vi "Format Http Request.vi"(0 "WS URI":string="ws://hostname.domain:80/resource/name", 2 "header string in":string, 3 "WebSocket Key":string="dKP/0gJzWzXMAh6SYdQ/sA==", 5 "error in":errorcluster, 9 "Relative URI Request (F)":bool) -> (16 "Http Request":string, 19 "error out":errorcluster)   [LabVIEW 2021, in "LV WebSockets.lvlib"]
uses:
  LV WebSockets.lvlib
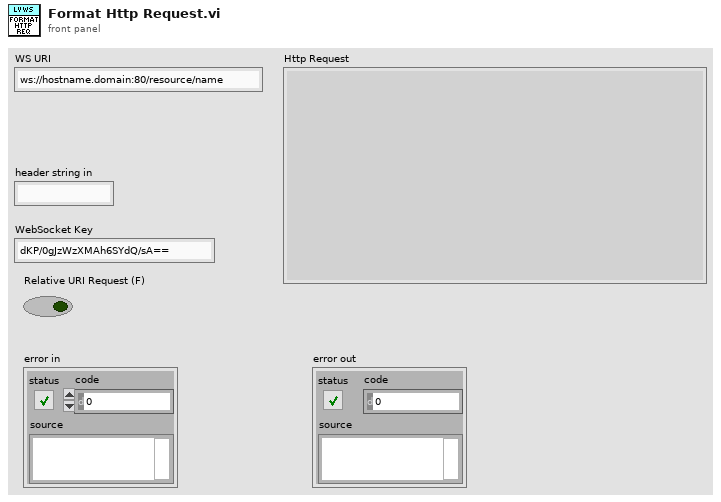
[diagram p1: front panel]
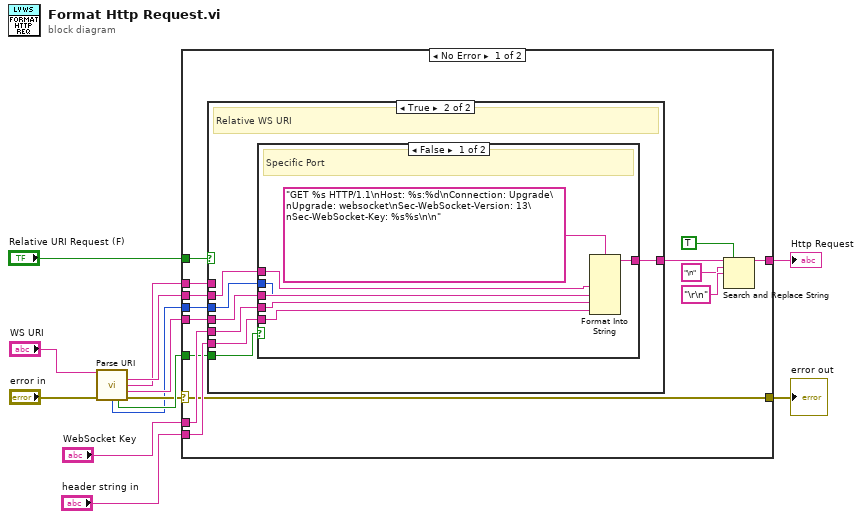
[diagram p0: block diagram]
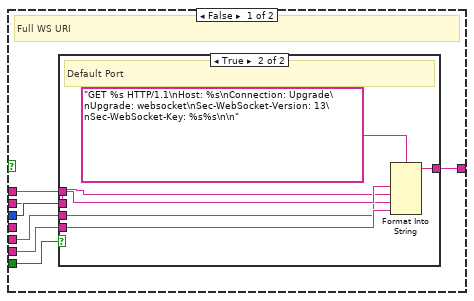
[diagram p2: hidden frame]
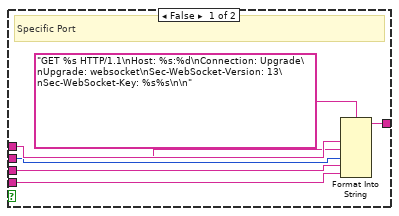
[diagram p3: hidden frame]
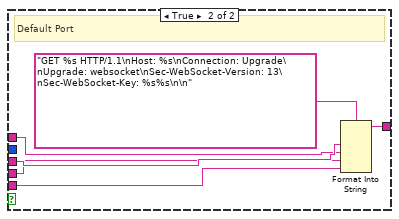
[diagram p4: hidden frame]
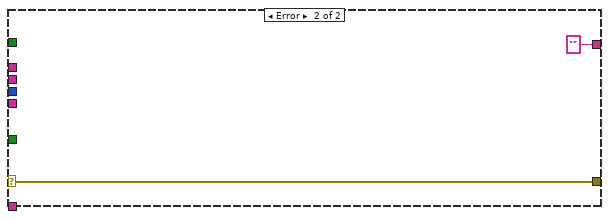
[diagram p5: hidden frame]
diagram:
  n1 = call "Parse URI.vi"("URI"="WS URI", "error in"="error in") -> ("Hostname"=w8:string, "HTTP URI"=w1:string, "Resource Name"=w3:string, "Port"=w2:u16, "Default Port"=w6:bool, "error out"=w5:errorcluster)  [unwired: 7 in, 1 out]
  n2 = case shown="No Error" w5 {
    selector: w5 -> [w15 w69]
    tunnel: "header string in" -> [w27 _]
    tunnel: "WebSocket Key" -> [w24 _]
    tunnel: [w22 "" ("result string")] -> w11
    tunnel: "Relative URI Request (F)" -> [w20 _]
    tunnel: w2 -> [w19 _]
    tunnel: w1 -> [w18 _]
    tunnel: w8 -> [w17 _]
    tunnel: w6 -> [w16 _]
    tunnel: [w15 w69] -> w4
    tunnel: w3 -> [w14 _]
    frame No Error {
      n3 = case shown="True" w20 {
        tunnel: w19 -> [w34 w50]
        tunnel: w18 -> [w33 _]
        tunnel: w27 -> [w32 w54]
        tunnel: w24 -> [w31 w53]
        tunnel: [w30 w52] -> w23
        tunnel: w17 -> [w28 w51]
        tunnel: w16 -> [w29 w49]
        tunnel: w14 -> [_ w48]
        frame False {
          # "Full WS URI"
          n4 = case shown="True" w29 {
            tunnel: w34 -> [w36 _]
            tunnel: w33 -> [w41 w47]
            tunnel: w32 -> [w40 w46]
            tunnel: w31 -> [w39 w45]
            tunnel: [w37 w43] -> w30
            tunnel: w28 -> [w35 w42]
            frame False {
              # "Specific Port"
              n5 = Format Into String(format string="GET %s HTTP/1.1\nHost: %s:%d\nConnection: Upgrade\nUpgrade: websocket\nSec-WebSocket-Version: 13\nSec-WebSocket-Key: %s%s\n\n", w41, w35, w36, w39, w40) -> (resulting string=w37:string)  [unwired: 2 in, 1 out]
            }
            frame True {
              # "Default Port"
              n6 = Format Into String(format string="GET %s HTTP/1.1\nHost: %s\nConnection: Upgrade\nUpgrade: websocket\nSec-WebSocket-Version: 13\nSec-WebSocket-Key: %s%s\n\n", w47, w42, w45, w46) -> (resulting string=w43:string)  [unwired: 2 in, 1 out]
            }
          }
        }
        frame True {
          # "Relative WS URI"
          n7 = case shown="False" w49 {
            tunnel: w48 -> [w61 w67]
            tunnel: w54 -> [w60 w66]
            tunnel: w53 -> [w59 w65]
            tunnel: [w57 w63] -> w52
            tunnel: w51 -> [w56 w62]
            tunnel: w50 -> [w55 _]
            frame False {
              # "Specific Port"
              n8 = Format Into String(format string="GET %s HTTP/1.1\nHost: %s:%d\nConnection: Upgrade\nUpgrade: websocket\nSec-WebSocket-Version: 13\nSec-WebSocket-Key: %s%s\n\n", w61, w56, w55, w59, w60) -> (resulting string=w57:string)  [unwired: 2 in, 1 out]
            }
            frame True {
              # "Default Port"
              n9 = Format Into String(format string="GET %s HTTP/1.1\nHost: %s\nConnection: Upgrade\nUpgrade: websocket\nSec-WebSocket-Version: 13\nSec-WebSocket-Key: %s%s\n\n", w67, w62, w65, w66) -> (resulting string=w63:string)  [unwired: 2 in, 1 out]
            }
          }
        }
      }
      n10 = Search and Replace String(replace all?=TRUE ("replace all? (F)"), input string=w23, search string="\n", replace string="\r\n" ("replace string (\"\")")) -> (result string=w22:string)  [unwired: 4 in, 3 out]
    }
    frame Error {
    }
  }
  "Http Request" <- w11
  "error out" <- w4
